vi "print Rx Packet Error.vi"(10 "error":u8, 11 "protocol_version":i32) -> ()   [LabVIEW 2016, in "dxl_x86_c.lvlib"]
doc: "WINDECLSPEC void printRxPacketError (int protocol_version, uint8_t error);"
uses:
  dxl_x86_c.lvlib
  dxl_x86_c.dll
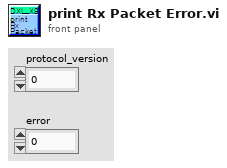
[diagram p1: front panel]
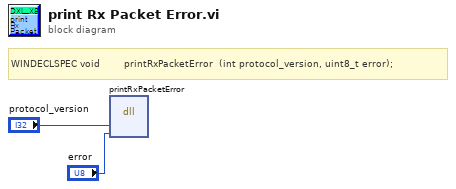
[diagram p0: block diagram]
diagram:
  # "WINDECLSPEC void        printRxPacketError  (int protocol_version, uint8_t error);"
  n1 = dll-call lib="C:/Users/Platform/Desktop/DynamixelSDK/labview/dxl_x86_c.lvlib/dxl_x86_c.*" fn="printRxPacketError"("protocol_version"="protocol_version", "error"="error") -> ()  [unwired: 6 in, 2 out]
